vi "ESIII EXO Gas Phase.vi"() -> ()   [LabVIEW 2012]
uses:
  <vilib>/Platform/TimedLoop/XDataNode/timing_clust.ctl
  <vilib>/Platform/TimedLoop/XDataNode/nitl_modes.ctl
  <vilib>/Platform/TimedLoop/XDataNode/wakeup.ctl
  <vilib>/addons/database/Connection.llb/DB Tools Open Connec (String).vi
  <vilib>/addons/database/Connection.llb/DB Tools Open Connec (Path).vi
  Labview_Spring2014/EXO200-LabView Dec.8/LabView Dec.8/SubVi's/DAQ Connection Variable.vi
  SubVi's/Connection Variable Common.vi
  Labview_Spring2014/Data grabber Folder/Documents and Settings/loaner/Desktop/Desktop/LabView Dec/LabView Dec.8/SubVi's/Plot Variable.vi
  SubVi's/Cryopump Variable.vi
  SubVi's/Monitor B Variable.vi
  Labview_Spring2014/EXO200-LabView Dec.8/LabView Dec.8/SubVi's/Time Zone Offset.vi
  Labview_Spring2014/EXO200-LabView Dec.8/LabView Dec.8/SubVi's/Time Variable.vi
  Labview_Spring2014/EXO200-LabView Dec.8/LabView Dec.8/SubVi's/Connection Variable 1.vi
  SubVi's/DAQ Data Variable.vi
  <vilib>/platform/TimedLoop/XDataNode/XDataNode.xnode
  <vilib>/Platform/TimedLoop/XDataNode/XDNodeRunTimeDep.lvlib
  Labview_Spring2014/SQL project lib.lvlib
  <vilib>/addons/database/NI_Database_API.lvlib
panel:
  out "Version out of date?":bool
  out "ESIII":bool
  in  "Info":bool
  in  "Quit Button":bool
  in  "Plot and Fit":bool
  in  "Cryopump Control":bool
  # "EXO 200"
  # "Release Date: 5/20/14"
  # "Control/Monitoring Programs"
  # "Database:"
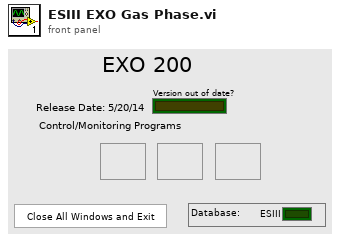
[diagram p1: front panel]
types:
  T1 = typedef "NI_Database_API.lvlib/Conn ObjectReference.ctl" = refnum<k1>
  T2 = typedef "XDNodeRunTimeDep.lvlib/timing_clust.ctl" = cluster{"Expected End [f-1]":u64, "Actual End [f-1]":u64, "Finished Late? [f-1]":bool, "Expected End [i-1]":u64, "Actual End [i-1]":u64, "Finished Late? [i-1]":bool, "Expected Start [i]":u64, "Actual Start [i]":u64, "Expected Start [f]":u64, "Actual Start [f]":u64, "Source Name":string, "Structure Name":string, "Period":i64, "Deadline":i64, "Offset":i64, "Start":i64, "Priority":i32, "Timeout":i32, "Mode":T3, "Wakeup Reason":T4, "Error":errorcluster, "Source Type":string, "Secondary Source Type":string, "Global End Time":u64, "Global Start Time":u64, "Frame Duration":u64, "Iteration Duration":u64, "Assigned CPU":i32, "I/O Scan Engine Mode":u32}
  T3 = typedef "XDNodeRunTimeDep.lvlib/nitl_modes.ctl" = enum32{"No Change", "Process missed periods, maintain original phase", "Discard missed periods, maintain original phase", "Process missed periods, ignore original phase", "Discard missed periods, ignore original phase"}
  T4 = typedef "XDNodeRunTimeDep.lvlib/wakeup.ctl" = enum32{"Normal", "Aborted", "Asynchronous wakeup", "Timing source error", "Timed loop error", "Timeout"}
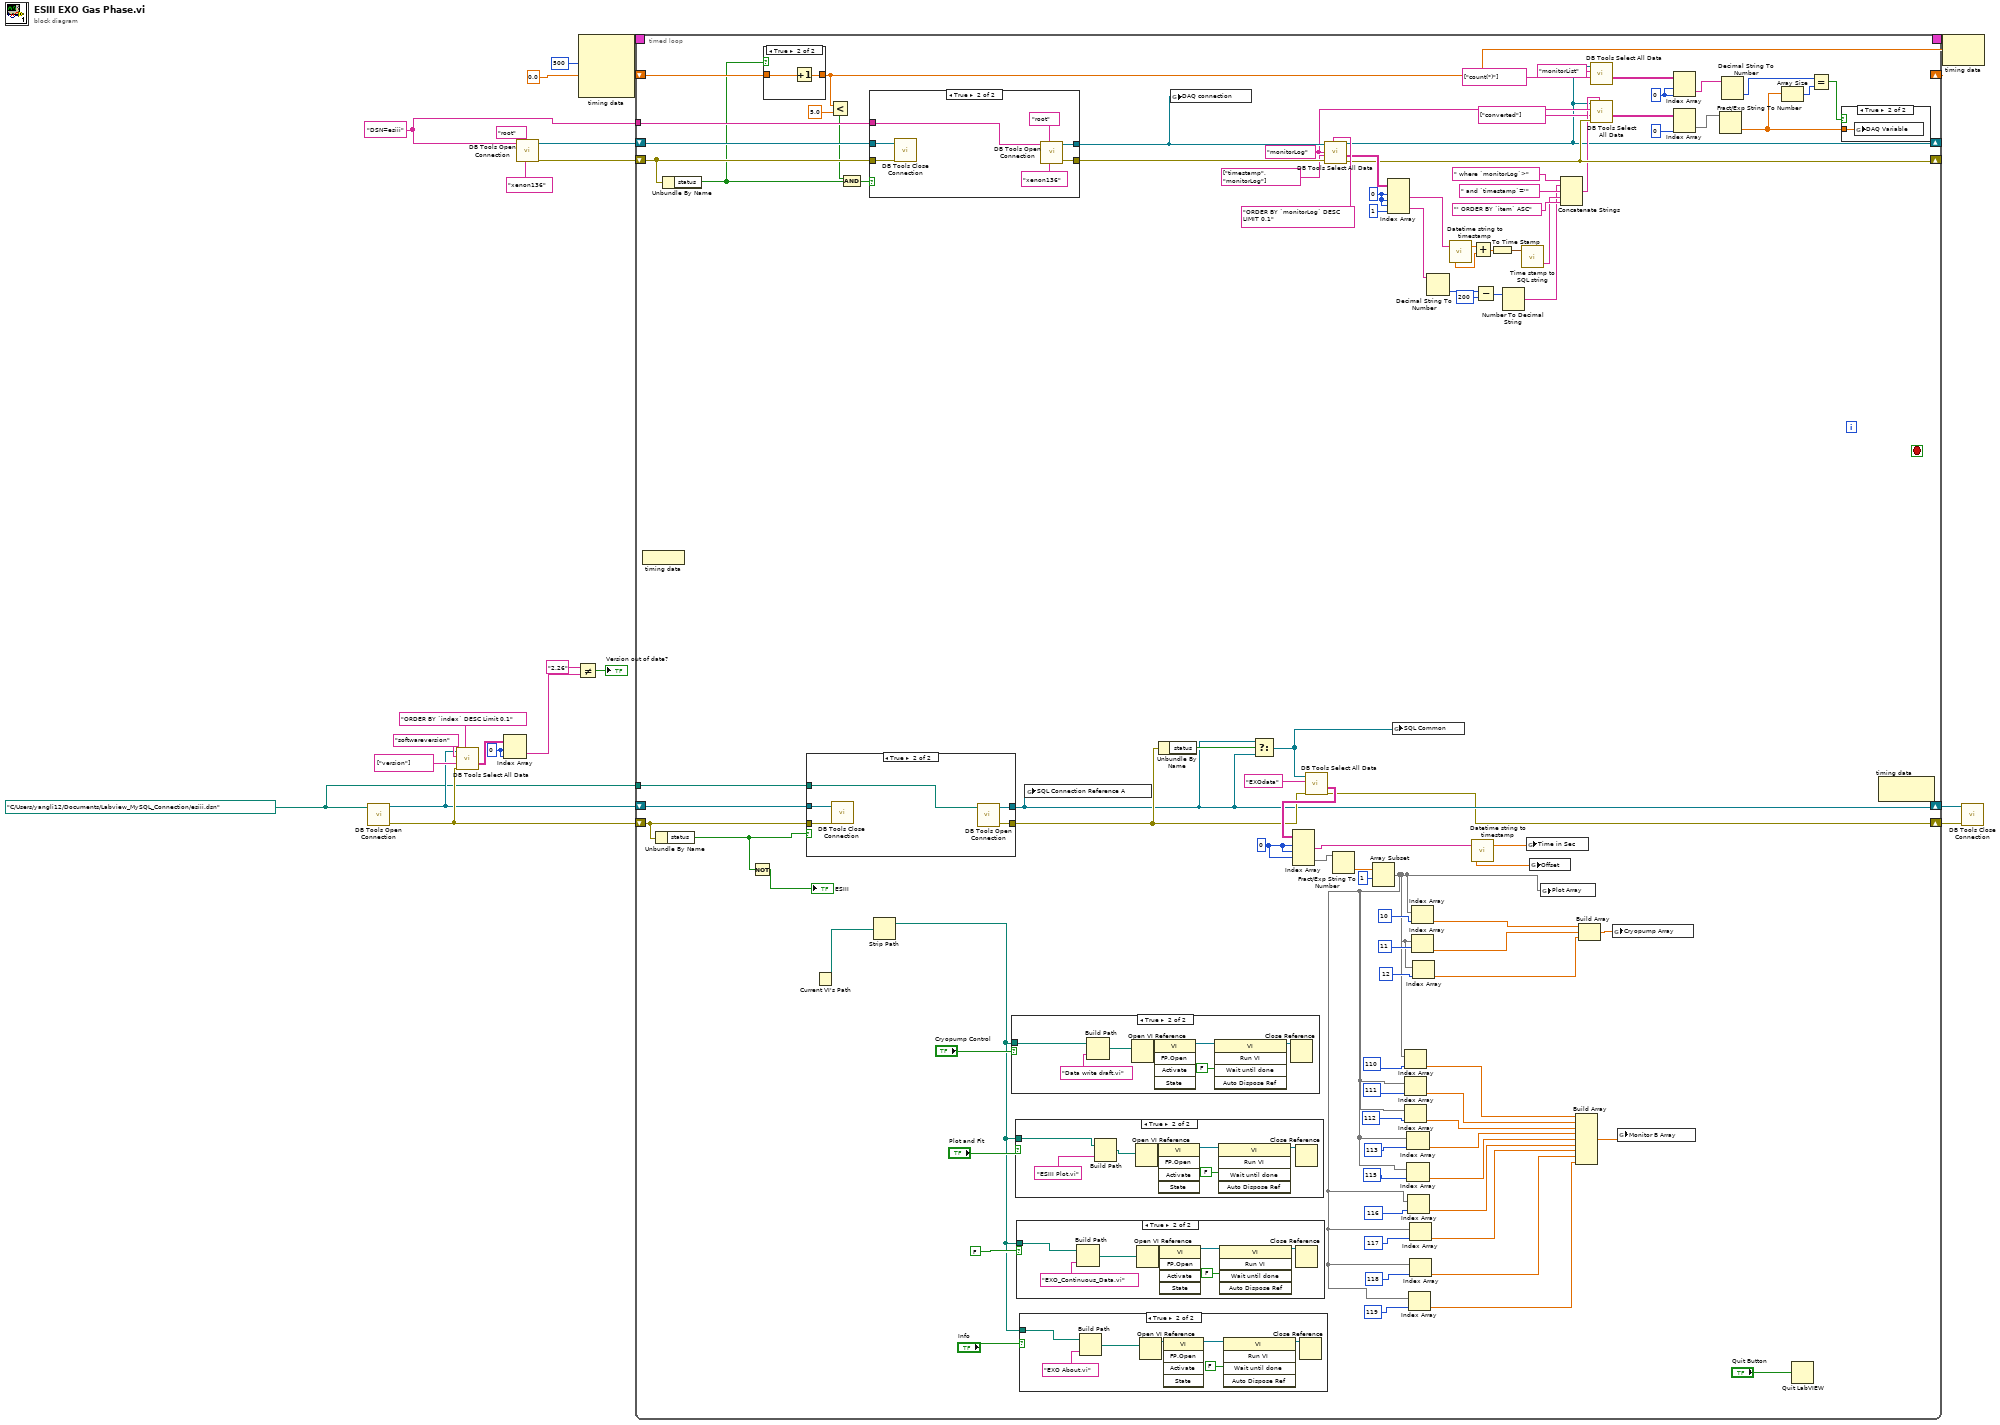
[diagram p0: block diagram]
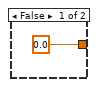
[diagram p2: hidden frame]
diagram:
  w1 = path "C:/Users/yangli12/Documents/Labview_MySQL_Connection/esiii.dsn" ("connection information")
  w4 = "DSN=esiii" ("userID")
  w9 = 0 ("index (row)")
  n1 = call-poly <vilib>:"DB Tools Open Connection.vi"("connection information"=w1) -> ("error out"=w17:errorcluster, "connection reference"=w5:T1)  [unwired: 4 in, 3 out]
  n2 = call <vilib>:"DB Tools Select All Data.vi"("optional clause"="ORDER BY `index` DESC Limit 0,1", "error in (no error)"=w17, "columns"=string[] ["version"], "table"="softwareversion", "connection reference"=w5) -> ("data"=w13:string[][])  [unwired: 3 out]
  n3 = Index Array(array=w13, index (row)=w9, index (col)=w9) -> (element=w11:string)
  n4 = call-poly <vilib>:"DB Tools Open Connection.vi"("password"="xenon136" ("userID"), "userID"="root", "connection information"=w4) -> ("error out"=w7:errorcluster, "connection reference"=w8:T1)  [unwired: 2 in, 3 out]
  n5 = Not Equal?(x="2.26", y=w11) -> (x != y?=→"Version out of date?":bool)
  n6 = node-c288(i64 500 ("Period")) -> (w22:T2)  [unwired: 3 out]
  n7 = timed-loop {
    timing: w22 -> [_]
    timing-out: [_] -> w21
    shift-right: [w37] -> w19
    shift-left: w5 -> [w112]
    shift-right: [w31] -> w18
    shift-left: w17 -> [w103]
    tunnel: w1 -> [w104]
    tunnel: w4 -> [w85]
    shift-right: [w52] -> _
    shift-left: w8 -> [w86]
    shift-right: [w77] -> _
    shift-left: w7 -> [w80]
    shift-right: [w39] -> _
    shift-left: 0.0 ("x+1") -> [w44]
    stop <- _ stop-if-true
    w48 = 0
    w64 = 0
    w76 = "monitorLog" ("table")
    w105 = 0 ("index (row)")
    n8 = node-c288 ("Output Node")() -> ()  [unwired: 1 out]
    n9 = Unbundle By Name(w103) -> ("status"=w90:bool)
    n10 = Unbundle By Name(w80) -> ("status"=w42:bool)
    n11 = Not(x=w90) -> (.not. x?=→"ESIII":bool)
    n12 = case shown="True" w42 {
      tunnel: [0.0 ("y") w125] -> w39
      tunnel: w44 -> [_ w124]
      frame False {
      }
      frame True {
        n13 = Increment(x=w124) -> (x+1=w125:dbl)
      }
    }
    n14 = case shown="True" w90 {
      tunnel: [w137 w142] -> w37
      tunnel: [w136 w141] -> w88
      tunnel: w112 -> [w137 w138]
      tunnel: w103 -> [w136 w139]
      tunnel: w104 -> [_ w140]
      frame False {
      }
      frame True {
        n15 = call <vilib>:"DB Tools Close Connection.vi"("error in (no error)"=w139, "connection reference"=w138) -> ()  [unwired: 6 out]
        n16 = call-poly <vilib>:"DB Tools Open Connection.vi"("connection information"=w140) -> ("error out"=w141:errorcluster, "connection reference"=w142:T1)  [unwired: 4 in, 3 out]
      }
    }
    n17 = Current VI's Path() -> (path=w114:path)
    n18 = Less?(x=w39, y=5.0) -> (x < y?=w40:bool)
    n19 = And(x=w40, y=w42) -> (x .and. y?=w43:bool)
    n20 = case shown="True" w43 {
      tunnel: [w128 w134] -> w82
      tunnel: [w127 w133] -> w81
      tunnel: w86 -> [w128 w130]
      tunnel: w80 -> [w127 w131]
      tunnel: w85 -> [_ w132]
      frame False {
      }
      frame True {
        n21 = call <vilib>:"DB Tools Close Connection.vi"("error in (no error)"=w131, "connection reference"=w130) -> ()  [unwired: 6 out]
        n22 = call-poly <vilib>:"DB Tools Open Connection.vi"("password"="xenon136" ("userID"), "userID"="root", "connection information"=w132) -> ("error out"=w133:errorcluster, "connection reference"=w134:T1)  [unwired: 2 in, 3 out]
      }
    }
    n23 = Strip Path(path=w114) -> (stripped path=w32:path)  [unwired: 1 out]
    n24 = case shown="True" "Cryopump Control" {
      tunnel: w32 -> [_ w166]
      frame False {
      }
      frame True {
        n25 = Build Path(base path=w166, name or relative path="Data write draft.vi") -> (appended path=w164:path)
        n26 = Open VI Reference(vi path=w164) -> (vi reference=w170:refnum<vi>)  [unwired: 2 in, 4 out]
        n27 = invoke class="VI" method="FP.Open"(reference=w170) -> (reference out=w169:refnum<vi>)  [unwired: 4 in, 4 out]
        n28 = invoke class="VI" method="Run VI"(reference=w169, "Wait until done"=FALSE ("Wait Until Done")) -> (reference out=w168:refnum<vi>)  [unwired: 3 in, 4 out]
        n29 = Close Reference(reference=w168) -> ()  [unwired: 1 in, 1 out]
      }
    }
    n30 = case shown="True" "Plot and Fit" {
      tunnel: w32 -> [_ w157]
      frame False {
      }
      frame True {
        n31 = Build Path(base path=w157, name or relative path="ESIII Plot.vi") -> (appended path=w158:path)
        n32 = Open VI Reference(vi path=w158) -> (vi reference=w163:refnum<vi>)  [unwired: 1 in, 5 out]
        n33 = invoke class="VI" method="FP.Open"(reference=w163) -> (reference out=w162:refnum<vi>)  [unwired: 4 in, 4 out]
        n34 = invoke class="VI" method="Run VI"(reference=w162, "Wait until done"=FALSE ("Wait Until Done")) -> (reference out=w160:refnum<vi>)  [unwired: 3 in, 4 out]
        n35 = Close Reference(reference=w160) -> ()  [unwired: 1 in, 1 out]
      }
    }
    n36 = case shown="True" FALSE {
      tunnel: w32 -> [_ w150]
      frame False {
      }
      frame True {
        n37 = Build Path(base path=w150, name or relative path="EXO_Continuous_Data.vi") -> (appended path=w151:path)
        n38 = Open VI Reference(vi path=w151) -> (vi reference=w156:refnum<vi>)  [unwired: 1 in, 5 out]
        n39 = invoke class="VI" method="FP.Open"(reference=w156) -> (reference out=w155:refnum<vi>)  [unwired: 4 in, 4 out]
        n40 = invoke class="VI" method="Run VI"(reference=w155, "Wait until done"=FALSE ("Wait Until Done")) -> (reference out=w154:refnum<vi>)  [unwired: 3 in, 4 out]
        n41 = Close Reference(reference=w154) -> ()  [unwired: 1 in, 1 out]
      }
    }
    n42 = case shown="True" "Info" {
      tunnel: w32 -> [_ w143]
      frame False {
      }
      frame True {
        n43 = Build Path(base path=w143, name or relative path="EXO About.vi") -> (appended path=w144:path)
        n44 = Open VI Reference(vi path=w144) -> (vi reference=w149:refnum<vi>)  [unwired: 1 in, 5 out]
        n45 = invoke class="VI" method="FP.Open"(reference=w149) -> (reference out=w148:refnum<vi>)  [unwired: 4 in, 4 out]
        n46 = invoke class="VI" method="Run VI"(reference=w148, "Wait until done"=FALSE ("Wait Until Done")) -> (reference out=w147:refnum<vi>)  [unwired: 3 in, 4 out]
        n47 = Close Reference(reference=w147) -> ()  [unwired: 1 in, 1 out]
      }
    }
    n48 = global write "Connection Variable 1.vi" "SQL Connection Reference A"(w37) -> ()
    n49 = Unbundle By Name(w88) -> ("status"=w99:bool)
    n50 = global write "DAQ Connection Variable.vi" "DAQ connection"(w82) -> ()
    n51 = Select(t=w37, s=w99, f=w37) -> (s? t:f=w89:T1)
    n52 = call <vilib>:"DB Tools Select All Data.vi"("error in (no error)"=w88, "table"="EXOdata", "connection reference"=w89) -> ("error out"=w31:errorcluster, "data"=w109:string[][])  [unwired: 2 in, 2 out]
    n53 = Index Array(array=w109, index (row) #1=w105, index (col) #1=w105, index (row) #2=w105) -> (element #1=w92:string, element #2=w106:string[])  [unwired: 1 in]
    n54 = call <vilib>:"DB Tools Select All Data.vi"("optional clause"="ORDER BY `monitorLog` DESC LIMIT 0,1", "error in (no error)"=w81, "columns"=string[] ["timestamp", "monitorLog"], "table"=w76, "connection reference"=w82) -> ("error out"=w77:errorcluster, "data"=w78:string[][], "connection reference out"=w52:T1)  [unwired: 1 out]
    n55 = Fract/Exp String To Number(string=w106) -> (number=w108:dbl[])  [unwired: 4 out]
    n56 = Array Subset(array=w108, index=1) -> (w23:dbl[])  [unwired: 1 in]
    n57 = Index Array(array=w78, index (row) #1=w64, index (col) #1=w64, index (row) #2=w64, index (col) #2=1 ("disabled index (col)")) -> (element #1=w68:string, element #2=w62:string)
    n58 = global write "Connection Variable Common.vi" "SQL Common"(w89) -> ()
    n59 = Index Array(array=w23, index=110) -> (element=w118:dbl)
    n60 = Index Array(array=w23, index=111) -> (element=w117:dbl)
    n61 = Index Array(array=w23, index=112) -> (element=w116:dbl)
    n62 = Index Array(array=w23, index=113) -> (element=w101:dbl)
    n63 = Index Array(array=w23, index=115 ("length")) -> (element=w97:dbl)
    n64 = Index Array(array=w23, index=116 ("length")) -> (element=w95:dbl)
    n65 = Index Array(array=w23, index=119) -> (element=w26:dbl)
    n66 = Index Array(array=w23, index=117) -> (element=w93:dbl)
    n67 = Index Array(array=w23, index=118) -> (element=w27:dbl)
    n68 = Index Array(array=w23, index=10 ("length")) -> (element=w34:dbl)
    n69 = Index Array(array=w23, index=11) -> (element=w87:dbl)
    n70 = Index Array(array=w23, index=12) -> (element=w24:dbl)
    n71 = Decimal String To Number(string=w62) -> (number=w61:i32)  [unwired: 3 out]
    n72 = call "Datetime string to timestamp.vi"("timestamp string"=w68) -> ("Time in sec"=w70:dbl, "Offset"=w65:dbl)  [unwired: 1 out]
    n73 = Add(x=w70, y=w65) -> (x+y=w66:dbl)
    n74 = call "Datetime string to timestamp.vi"("timestamp string"=w92) -> ("Time in sec"=w91:dbl, "Offset"=w30:dbl)  [unwired: 1 out]
    n75 = Subtract(x=w61, y=200) -> (x-y=w58:i32)
    n76 = To Time Stamp(1:w66) -> (0:w69:timestamp)
    n77 = Number To Decimal String(number=w58) -> (decimal integer string=w57:string)  [unwired: 1 out]
    n78 = call "Time stamp to SQL string.vi"("time stamp"=w69) -> ("SQL format date-time string"=w67:string)  [unwired: 1 in, 1 out]
    n79 = global write "Time Variable.vi" "Time in Sec"(w91) -> ()
    n80 = global write "Time Zone Offset.vi" "Offset"(w30) -> ()
    n81 = global write "Plot Variable.vi" "Plot Array"(w23) -> ()
    n82 = Concatenate Strings(" where `monitorLog`>" ("optional clause"), w57, " and `timestamp`='" ("optional clause"), w67, "' ORDER BY `item` ASC" ("optional clause")) -> (w73:string)
    n83 = Build Array(w118, w117, w116, w101, w97, w95, w93, w27, w26) -> (w35:dbl[])
    n84 = Build Array(w34, w87, w24) -> (w36:dbl[])
    n85 = call <vilib>:"DB Tools Select All Data.vi"("columns"=string[] ["count(*)"], "table"="monitorList", "connection reference"=w52) -> ("data"=w49:string[][])  [unwired: 1 in, 4 out]
    n86 = call <vilib>:"DB Tools Select All Data.vi"("optional clause"=w73, "error in (no error)"=w77, "columns"=string[] ["converted"], "table"=w76, "connection reference"=w52) -> ("data"=w71:string[][])  [unwired: 3 out]
    n87 = global write "Cryopump Variable.vi" "Cryopump Array"(w36) -> ()
    n88 = global write "Monitor B Variable.vi" "Monitor B Array"(w35) -> ()
    n89 = Index Array(array=w49, index (row)=w48, index (col)=w48) -> (element=w47:string)
    n90 = Index Array(array=w71, index (col)=0) -> (element=w83:string[])  [unwired: 1 in]
    n91 = Fract/Exp String To Number(string=w83) -> (number=w55:dbl[])  [unwired: 4 out]
    n92 = Decimal String To Number(string=w47) -> (number=w46:i32)  [unwired: 3 out]
    n93 = Array Size(array=w55) -> (size(s)=w54:i32)
    n94 = Quit LabVIEW(quit? (T)="Quit Button") -> ()
    n95 = Equal?(x=w46, y=w54) -> (x = y?=w53:bool)
    n96 = case shown="True" w53 {
      tunnel: w55 -> [_ w126]
      frame False {
      }
      frame True {
        n97 = global write "DAQ Data Variable.vi" "DAQ Variable"(w126) -> ()
      }
    }
    n98 = node-c288() -> ()  [unwired: 2 out]
  }
  n99 = node-c288(w21) -> ()  [unwired: 1 out]
  n100 = call <vilib>:"DB Tools Close Connection.vi"("error in (no error)"=w18, "connection reference"=w19) -> ()  [unwired: 6 out]
